vi "JSON Parse Channel Number.vi"(11 "device string":string) -> (0 "error out":errorcluster, 2 "Device Subtype":string, 3 "Channel":i32)   [LabVIEW 2019]
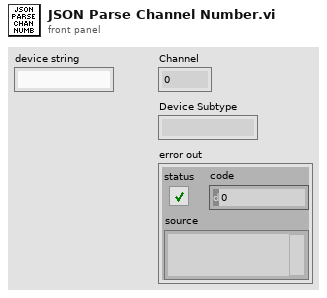
[diagram p1: front panel]
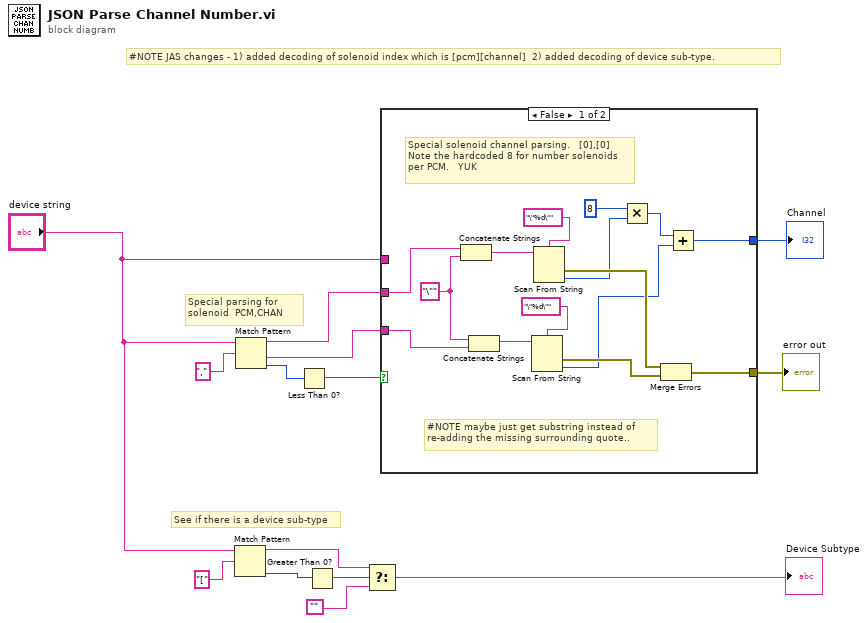
[diagram p0: block diagram]
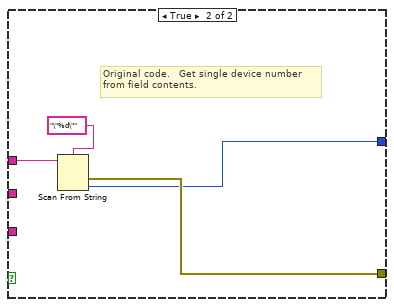
[diagram p2: hidden frame]
diagram:
  # "See if there is a device sub-type"
  # "#NOTE JAS changes - 1) added decoding of solenoid index which is [pcm][channel]  2) added decoding of device sub-type."
  # "Special parsing for\nsolenoid  PCM,CHAN"
  n1 = Match Pattern(string="device string", regular expression="[") -> (before substring=w4:string, offset past match=w5:i32)  [unwired: 1 in, 2 out]
  n2 = Match Pattern(string="device string", regular expression=",") -> (before substring=w8:string, after substring=w9:string, offset past match=w13:i32)  [unwired: 1 in, 1 out]
  n3 = Less Than 0?(x=w13) -> (x < 0?=w12:bool)
  n4 = Greater Than 0?(x=w5) -> (x > 0?=w2:bool)
  n5 = Select(t=w4, s=w2, f="") -> (s? t:f=→"Device Subtype":string)
  n6 = case shown="False" w12 {
    tunnel: [w27 w32] -> w11
    tunnel: [w24 w31] -> w10
    tunnel: "device string" -> [_ w30]
    tunnel: w8 -> [w19 _]
    tunnel: w9 -> [w17 _]
    frame False {
      w18 = "\"" ("string")
      # "#NOTE maybe just get substring instead of \nre-adding the missing surrounding quote.."
      # "Special solenoid channel parsing.   [0],[0]\nNote the hardcoded 8 for number solenoids per PCM.   YUK"
      n7 = Concatenate Strings(w19, w18) -> (w15:string)
      n8 = Concatenate Strings(w18, w17) -> (w16:string)
      n9 = Scan From String(format string="\"%d\"", input string=w16) -> (error out=w26:errorcluster, output 1=w23:i32)  [unwired: 3 in, 2 out]
      n10 = Scan From String(format string="\"%d\"", input string=w15) -> (error out=w25:errorcluster, output 1=w22:i32)  [unwired: 3 in, 2 out]
      n11 = Multiply(x=8, y=w22) -> (x*y=w21:i32)
      n12 = Merge Errors(w25, w26) -> (w27:errorcluster)
      n13 = Add(x=w21, y=w23) -> (x+y=w24:i32)
    }
    frame True {
      # "Original code.   Get single device number\nfrom field contents."
      n14 = Scan From String(format string="\"%d\"", input string=w30) -> (error out=w32:errorcluster, output 1=w31:i32)  [unwired: 3 in, 2 out]
    }
  }
  "error out" <- w11
  "Channel" <- w10
